vi "Set All Parameters.vi"(8 "error in (no error)":errorcluster, 10 "Parameters":T1={"Type"=enum."Mouse Move", "X"=0, "Y"=0, "Delay"=0, "Key"=65, "Repeat"=0, "RClick?"=FALSE, "App/Window Name"="", "Notes"="", "Assertion Type"=enum."Control Position", "Control Name"="", "Disabled"=enum."Enabled", "Visible"=enum."Visible", "Left"=0, "Top"=0, "Width"=0, "Height"=0, "Expected Image"={"image type"=0, "image depth"=0, "image"=[], "mask"=[], "colors"=[], "Rectangle"={"left"=0, "top"=0, "right"=0, "bottom"=0}}}, 11 "Keyboard Macro in":refnum<class "Keyboard Macro.lvclass">) -> (0 "error out":errorcluster, 3 "Keyboard Macro out":refnum<class "Keyboard Macro.lvclass">)   [LabVIEW 2020, in "MacroAssert.lvlib" / "Keyboard Macro.lvclass"]
uses:
  Keyboard Macro.lvclass
  Keyboard Macro.lvclass/Keyboard Macro.ctl
  Macro Step/Macro Step.lvclass
  CTLs/Step Type V3.ctl
  MacroAssert.lvlib
  CTLs/Assertion Type.ctl
  <vilib>/picture/picture.llb/imagedata.ctl
  CTLs/Step V3.ctl
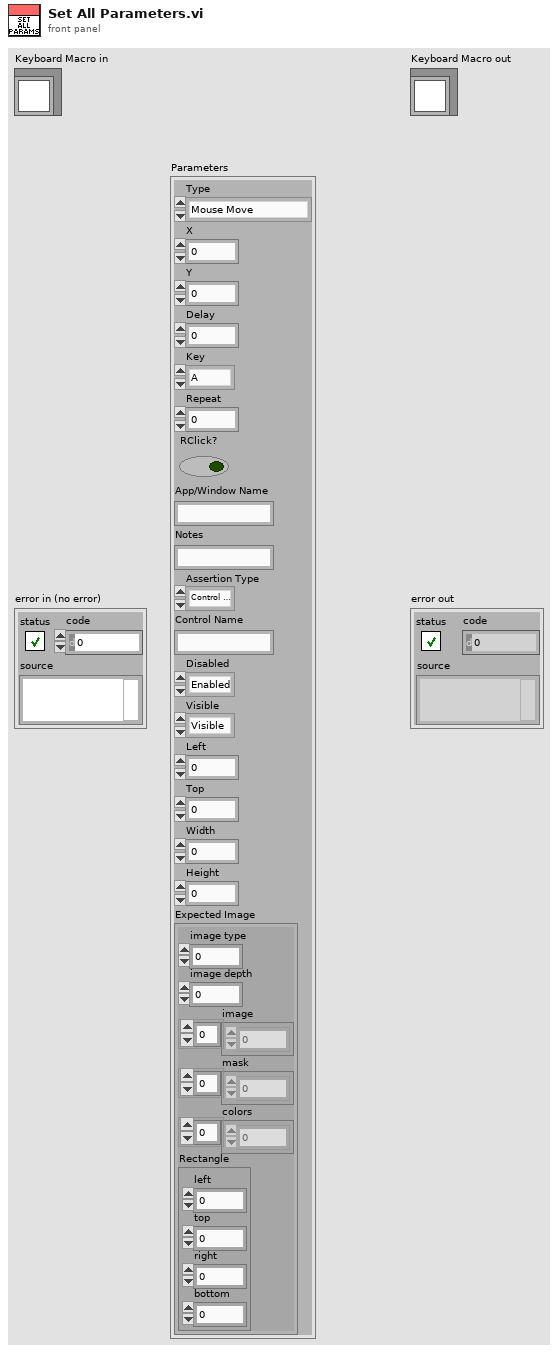
[diagram p1: front panel]
types:
  T1 = typedef "MacroAssert.lvlib/Step V3.ctl" = cluster{"Type":T2, "X":i32, "Y":i32, "Delay":i32, "Key":u8, "Repeat":i32, "RClick?":bool, "App/Window Name":string, "Notes":string, "Assertion Type":T3, "Control Name":string, "Disabled":enum8{"Enabled", "Disabled", "Disabled and Grayed Out"}, "Visible":enum16{"Visible", "Not Visible"}, "Left":i16, "Top":i16, "Width":i16, "Height":i16, "Expected Image":T4}
  T2 = typedef "MacroAssert.lvlib/Step Type V3.ctl" = enum16{"Mouse Move", "Mouse Click", "Key Press", "Wait", "Mouse Down", "Mouse Up", "Key Down", "Key Up", "Test Assertion", "Maximize Window", "Restore Window", "Minimize Window", "Close Window", "Bring Window to Front", "Send Window to Back"}
  T3 = typedef "MacroAssert.lvlib/Assertion Type.ctl" = enum16{"Control Position", "Control Visible", "Control Disabled", "Control Image"}
  T4 = typedef "imagedata.ctl" = cluster{"image type":i32, "image depth":i32, "image":u8[], "mask":u8[], "colors":u32[], "Rectangle":cluster{"left":i16, "top":i16, "right":i16, "bottom":i16}}
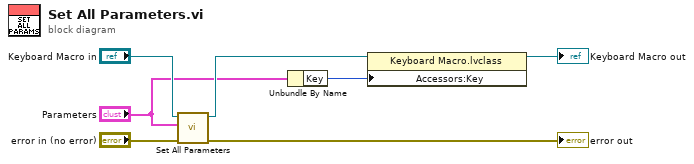
[diagram p0: block diagram]
diagram:
  n1 = call-parent "Set All Parameters.vi"("error in (no error)"="error in (no error)", "Parameters"="Parameters", "Macro Step in"="Keyboard Macro in") -> ("error out"=→"error out":errorcluster, "Macro Step out"=w6:refnum<class "Keyboard Macro.lvclass">)  [unwired: 7 in]
  n2 = Unbundle By Name("Parameters") -> ("Key"=w1:u8)
  n3 = property class="Keyboard Macro.lvclass"(reference=w6, "Accessors:Key"=w1) -> (reference out=→"Keyboard Macro out":refnum<class "Keyboard Macro.lvclass">)  [unwired: 1 in, 1 out]
